vi "FTW-Project-Filepath.vi"(0 "Project Ref":refnum<vi>, 11 "error in":errorcluster) -> (4 "Project Ref out":refnum<vi>, 6 "Project Filepath":path, 8 "Project Directory":path, 15 "error out":errorcluster)   [LabVIEW 2012]
panel:
  # "Inputs"
  # "Outputs"
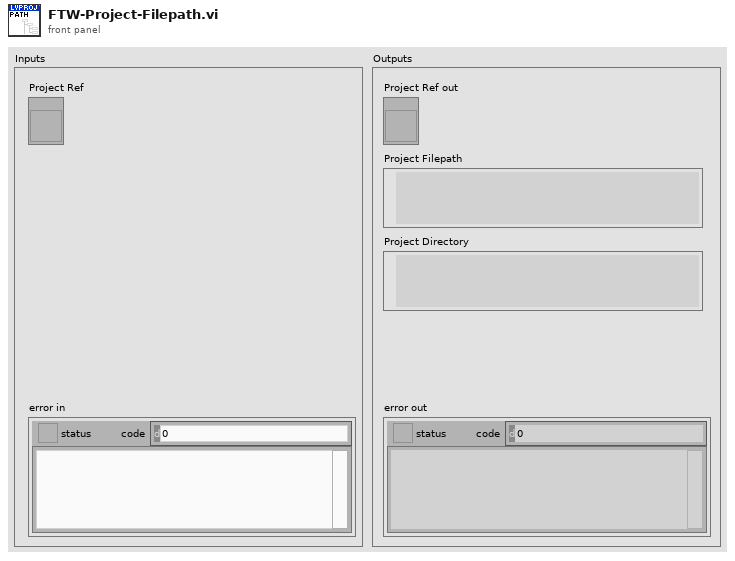
[diagram p1: front panel]
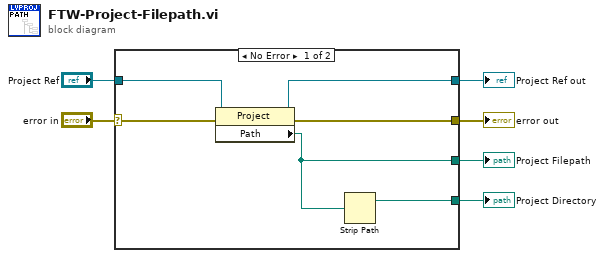
[diagram p0: block diagram]
diagram:
  n1 = case shown="No Error" "error in" {
    selector: "error in" -> [w10 w14]
    tunnel: [w9 w14] -> w6
    tunnel: "Project Ref" -> [w11 w13]
    tunnel: [w12 w13] -> w3
    tunnel: [w8 _] -> w2
    tunnel: [w7 _] -> w1
    frame No Error {
      n2 = property class="Project"(reference=w11, error in=w10) -> (reference out=w12:refnum<vi>, error out=w9:errorcluster, "Path"=w8:path)
      n3 = Strip Path(path=w8) -> (stripped path=w7:path)  [unwired: 1 out]
    }
    frame Error {
    }
  }
  "error out" <- w6
  "Project Ref out" <- w3
  "Project Filepath" <- w2
  "Project Directory" <- w1
